vi "Write Edit Time Configuration.vi"(8 "error in (no error)":errorcluster, 10 "Edit Time Configuration":string, 11 "Session in":refnum<class "Plugin Session.lvclass">) -> (0 "error out":errorcluster, 3 "Session out":refnum<class "Plugin Session.lvclass">)   [LabVIEW 2023, in "InstrumentStudio Plugin SDK.lvlib" / "Plugin Session.lvclass"]
doc: "Call this VI to update the edit-time configuration string for your plugin panel."
uses:
  Plugin Session.lvclass
  Plugin Session.lvclass/Plugin Session.ctl
  Read Session Id.vi
  NationalInstruments.VIHost.Interop.dll
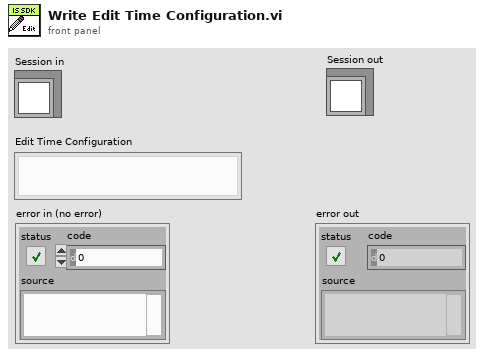
[diagram p1: front panel]
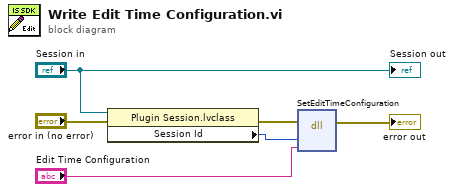
[diagram p0: block diagram]
diagram:
  n1 = property class="Plugin Session.lvclass"(reference="Session in", error in="error in (no error)") -> (error out=w6:errorcluster, "Session Id"=w2:u64)  [unwired: 1 out]
  n2 = dll-call lib="C:/Users/nmurphy/Downloads/InstrumentStudio_LabVIEW_Plugins/LabVIEW/ExampleProject/PluginSDK/NationalInstruments.VIHost.Interop.dll" fn="SetEditTimeConfiguration"(error in=w6, "hostId"=w2, "configuration"="Edit Time Configuration") -> (error out=→"error out":errorcluster)  [unwired: 5 in, 1 out]
  "Session out" <- "Session in"
